vi "save_all_signal.vi"(8 "error in (no error)":errorcluster, 9 "Variable Names Array":string[](array[string]), 10 "# of points":u32[](array[numeric]), 11 "file path":path) -> (0 "error out":errorcluster)   [LabVIEW 2013]
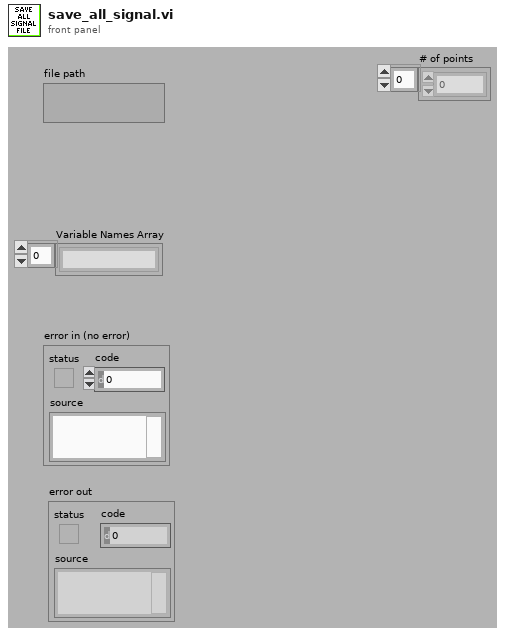
[diagram p1: front panel]
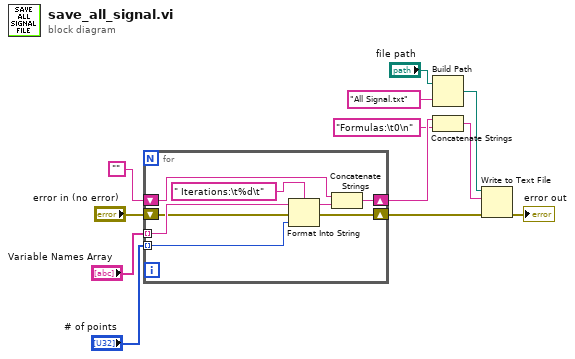
[diagram p0: block diagram]
diagram:
  n1 = for {
    tunnel: "Variable Names Array" -> [w20] mode=indexing
    tunnel: "# of points" -> [w18] mode=indexing
    shift-right: [w17] -> w7
    shift-left: "" -> [w15]
    shift-right: [w14] -> w4
    shift-left: "error in (no error)" -> [w13]
    n2 = Format Into String(format string=" Iterations:\t%d\t", initial string=w20, error in=w13, w18) -> (resulting string=w16:string, error out=w14:errorcluster)
    n3 = Concatenate Strings(w15, w16) -> (w17:string)
  }
  n4 = Build Path(base path="file path", name or relative path="All Signal.txt") -> (appended path=w1:path)
  n5 = Concatenate Strings(w7, "Formulas:\t0\n" ("string")) -> (w5:string)
  n6 = Write to Text File(file (use dialog)=w1, text=w5, error in=w4) -> (error out=→"error out":errorcluster)  [unwired: 1 in, 2 out]
